vi "Switch.vi"(2 "threshold":dbl=1.0 format="%.2f", 3 "input point 2":dbl format="%.2f", 4 "control input":dbl format="%.2f", 5 "input point 1":dbl format="%.2f") -> (1 "output point":dbl format="%.2f")   [LabVIEW 2020, in "NI_AdvCtrl_nonlinear.lvlib"]
doc: "LabVIEW no longer supports this VI. You can obtain similar functionality by installing the LabVIEW Simulation Module.\n\nSwitches between two values. It is output=input point 1 in case of control input>threshold and output=input point 2 otherwise."
uses:
  <vilib>/addons/control/advanced/NI_AdvCtrl_nonlinear.lvlib
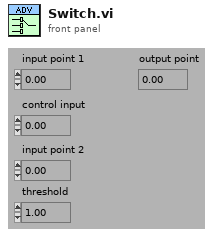
[diagram p1: front panel]
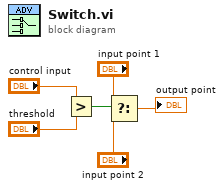
[diagram p0: block diagram]
diagram:
  n1 = Greater?(x="control input", y="threshold") -> (0:w3:bool)
  n2 = Select(t="input point 1", s=w3, f="input point 2") -> (s? t:f=→"output point":dbl)
